vi "Maxi Gauge-Display control.vi"(0 "VISA-Ressource in":refnum<visa-resource-name>, 1 "W/R":bool, 5 "Node address":i8=-1 min=-1 max=31 step=1, 7 "Set Contrast":i8=-1 min=-1 max=20 step=1, 9 "Set Screensave":i8=-1 min=-1 max=99 step=1, 11 "Fehler (Eingang)":errorcluster) -> (4 "VISA-Ressource out":refnum<visa-resource-name>, 8 "Get Contrast":i8=-1 min=-1 max=20 step=1, 10 "Get Screensave":i8=-1 min=-1 max=99 step=1, 15 "Fehler (Ausgang)":errorcluster)   [LabVIEW 2013, in "Maxi Gauge.lvlib"]
uses:
  <instrlib>/Maxi Gauge/Maxi Gauge.lvlib
panel:
  # "h"
  # "h"
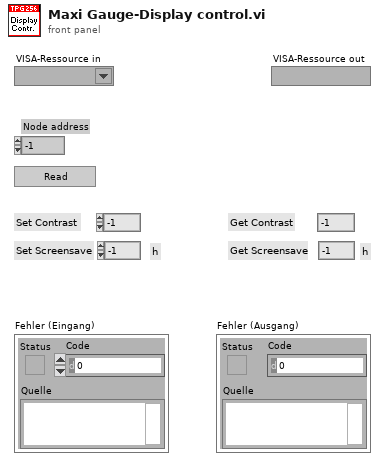
[diagram p1: front panel]
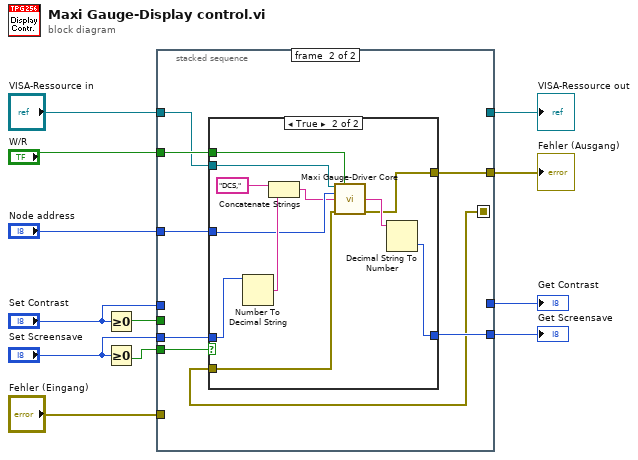
[diagram p0: block diagram]
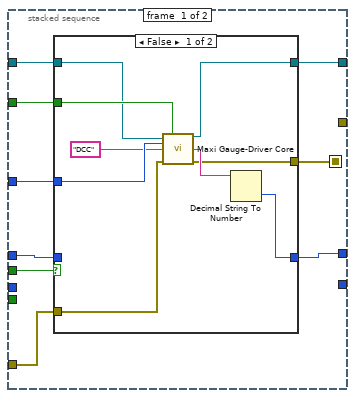
[diagram p2: hidden frame]
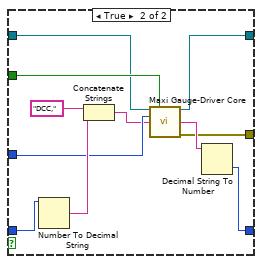
[diagram p3: hidden frame]
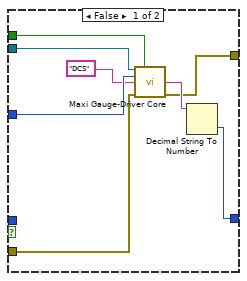
[diagram p4: hidden frame]
diagram:
  n1 = Greater Or Equal To 0?(x="Set Contrast") -> (x >= 0?=w6:bool)
  n2 = Greater Or Equal To 0?(x="Set Screensave") -> (x >= 0?=w5:bool)
  n3 = stacked-sequence {
    seq-local: [w13 _] -> [_ w42]
    tunnel: "W/R" -> [w21 w49]
    tunnel: [w20 _] -> w9
    tunnel: w6 -> [w19 _]
    tunnel: "Set Contrast" -> [w18 _]
    tunnel: w5 -> [_ w48]
    tunnel: "Set Screensave" -> [_ w47]
    tunnel: [_ w46] -> w8
    tunnel: [_ w45] -> w1
    tunnel: "Node address" -> [w17 w44]
    tunnel: "VISA-Ressource in" -> [w16 w43]
    tunnel: [w15 _] -> w3
    tunnel: "Fehler (Eingang)" -> [w14 _]
    frame #0 {
      n4 = case shown="False" w19 {
        tunnel: w21 -> [w29 w40]
        tunnel: [w28 w37] -> w20
        tunnel: w18 -> [_ w36]
        tunnel: [w27 w35] -> w13
        tunnel: w17 -> [w26 w34]
        tunnel: w16 -> [w24 w32]
        tunnel: [w23 w31] -> w15
        tunnel: w14 -> [w22 _]
        frame False {
          n5 = call <instrlib>:"Maxi Gauge-Driver Core.vi"("VISA-Ressource in"=w24, "Write/Read"=w29, "Node address"=w26, "Command"="DCC", "Fehler (Eingang)"=w22) -> ("VISA-Ressource out"=w23:refnum<visa-resource-name>, "String Out"=w30:string, "Fehler (Ausgang)"=w27:errorcluster)  [unwired: 8 in]
          n6 = Decimal String To Number(string=w30) -> (number=w28:i32)  [unwired: 2 in, 1 out]
        }
        frame True {
          n7 = Number To Decimal String(number=w36) -> (decimal integer string=w39:string)  [unwired: 1 in]
          n8 = Concatenate Strings("DCC,", w39) -> (w33:string)
          n9 = call <instrlib>:"Maxi Gauge-Driver Core.vi"("VISA-Ressource in"=w32, "Write/Read"=w40, "Node address"=w34, "Command"=w33) -> ("VISA-Ressource out"=w31:refnum<visa-resource-name>, "String Out"=w41:string, "Fehler (Ausgang)"=w35:errorcluster)  [unwired: 9 in]
          n10 = Decimal String To Number(string=w41) -> (number=w37:i32)  [unwired: 2 in, 1 out]
        }
      }
    }
    frame #1 {
      n11 = case shown="True" w48 {
        tunnel: w49 -> [w56 w67]
        tunnel: [w55 w64] -> w46
        tunnel: w47 -> [_ w63]
        tunnel: [w54 w62] -> w45
        tunnel: w44 -> [w53 w61]
        tunnel: w43 -> [w51 w59]
        tunnel: w42 -> [w50 w58]
        frame False {
          n12 = call <instrlib>:"Maxi Gauge-Driver Core.vi"("VISA-Ressource in"=w51, "Write/Read"=w56, "Node address"=w53, "Command"="DCS", "Fehler (Eingang)"=w50) -> ("String Out"=w57:string, "Fehler (Ausgang)"=w54:errorcluster)  [unwired: 8 in, 1 out]
          n13 = Decimal String To Number(string=w57) -> (number=w55:i32)  [unwired: 2 in, 1 out]
        }
        frame True {
          n14 = Number To Decimal String(number=w63) -> (decimal integer string=w66:string)  [unwired: 1 in]
          n15 = Concatenate Strings("DCS,", w66) -> (w60:string)
          n16 = call <instrlib>:"Maxi Gauge-Driver Core.vi"("VISA-Ressource in"=w59, "Write/Read"=w67, "Node address"=w61, "Command"=w60, "Fehler (Eingang)"=w58) -> ("String Out"=w68:string, "Fehler (Ausgang)"=w62:errorcluster)  [unwired: 8 in, 1 out]
          n17 = Decimal String To Number(string=w68) -> (number=w64:i32)  [unwired: 2 in, 1 out]
        }
      }
    }
  }
  "Get Contrast" <- w9
  "Get Screensave" <- w8
  "VISA-Ressource out" <- w3
  "Fehler (Ausgang)" <- w1
